vi "Remove NaN(1D).vi"(10 "Index":i32, 11 "Input":dbl[](array[numeric])) -> (3 "Numeric":dbl)   [LabVIEW 2019, in "Zen Analytics.lvlib" / "Zen Analytics.lvclass"]
uses:
  Zen Analytics.lvclass
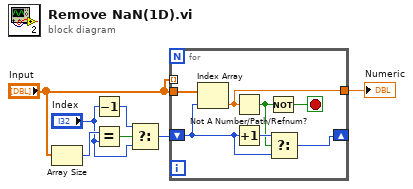
[diagram p0: block diagram]
diagram:
  n1 = Array Size(array="Input") -> (size(s)=w5:i32)
  n2 = Decrement(x="Index") -> (x-1=w3:i32)
  n3 = Equal?(x=w5, y="Index") -> (x = y?=w4:bool)
  n4 = Select(t=w3, s=w4, f="Index") -> (s? t:f=w1:i32)
  n5 = for {
    tunnel: "Input" -> [w12]
    tunnel: [w9] -> w7
    shift-right: [w13] -> _
    shift-left: w1 -> [w11]
    tunnel: "Input" -> [_] mode=indexing
    stop <- w8 stop-if-true
    n6 = Index Array(array=w12, index=w11) -> (element=w9:dbl)
    n7 = Not A Number/Path/Refnum?(number/path/refnum=w9) -> (NaN/Path/Refnum?=w10:bool)
    n8 = Increment(x=w11) -> (x+1=w14:i32)
    n9 = Not(x=w10) -> (.not. x?=w8:bool)
    n10 = Select(t=w14, s=w10, f=w11) -> (s? t:f=w13:i32)
  }
  "Numeric" <- w7
